vi "Remove NIPKG By Name.vi"(0 "package to remove":string, 11 "error in":errorcluster) -> (4 "standard output":string, 15 "error out":errorcluster)   [LabVIEW 2020]
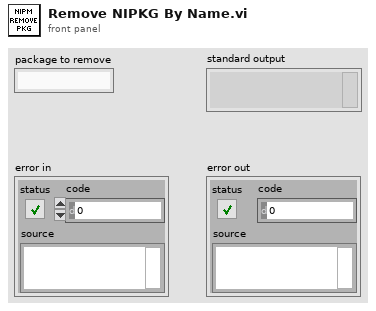
[diagram p1: front panel]
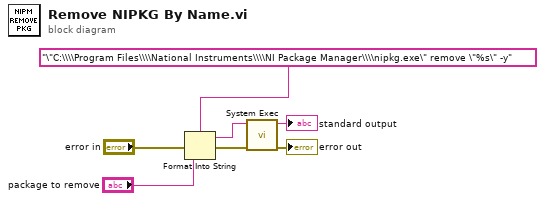
[diagram p0: block diagram]
diagram:
  n1 = Format Into String(format string="\"C:\\\\Program Files\\\\National Instruments\\\\NI Package Manager\\\\nipkg.exe\" remove \"%s\" -y", error in="error in", "package to remove") -> (resulting string=w3:string, error out=w4:errorcluster)  [unwired: 1 in]
  n2 = call <vilib>:"System Exec.vi"("error in (no error)"=w4, "command line"=w3) -> ("error out"=→"error out":errorcluster, "standard output"=→"standard output":string)  [unwired: 6 in, 2 out]
